vi "年与天换算.vi"() -> ()   [LabVIEW 2020]
doc: "本VI是为《我和LabVIEW》一书编写的示例。\n关于本书的介绍请参考网页：\nhttp://ruanqizhen.spaces.live.com/blog/cns!5852D4F797C53FB6!4310.entry"
panel:
  out "天":dbl[unit]
  in  "年":dbl[unit]
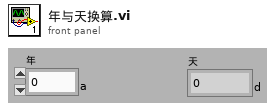
[diagram p1: front panel]
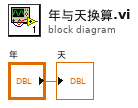
[diagram p0: block diagram]
diagram:
  "天" <- "年"
